vi "Read Exe Version.vi"() -> (2 "String":string, 3 "FileVersion":string)   [LabVIEW 2020]
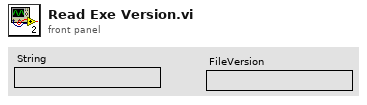
[diagram p1: front panel]
types:
  T1 = enum32{"invalid app kind", "Development System", "Run Time System", "Student Edition", "Embedded LabVIEW", "Evaluation", "Custom"}
  T2 = typedef "FileVersionInformation.ctl" = cluster{"FileVersion":string, "ProductName":string, "InternalName":string, "CompanyName":string, "LegalCopyright":string, "FileDescription":string}
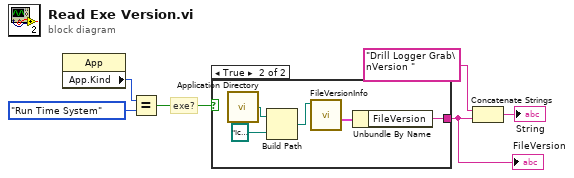
[diagram p0: block diagram]
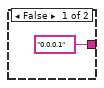
[diagram p2: hidden frame]
diagram:
  # "exe?"
  n1 = property class="App"() -> ("App.Kind"=w3:T1)  [unwired: 2 in, 2 out]
  n2 = Equal?(x=w3, y=T1."Run Time System" ("Application:Kind")) -> (x = y?=w5:bool)
  n3 = case shown="True" w5 {
    tunnel: ["0.0.0.1" ("FileVersion") w11] -> w6
    frame False {
    }
    frame True {
      n4 = call <vilib>:"Application Directory.vi"() -> ("Application Directory"=w10:path)
      n5 = Build Path(base path=w10, name or relative path=path "Ice Nucleation.exe") -> (appended path=w9:path)
      n6 = call <vilib>:"FileVersionInfo.vi"("Application Path in"=w9) -> ("FileVersionInfo Out"=w12:T2)  [unwired: 7 in, 3 out]
      n7 = Unbundle By Name(w12) -> ("FileVersion"=w11:string)
    }
  }
  "FileVersion" <- w6
  n8 = Concatenate Strings("Drill Logger Grab\nVersion " ("Version"), w6) -> (→"String":string)
